vi "FlatToRichcif_plugincore_PluginNames.vi"(5 "OutputClusterType":T1, 11 "InputCluster":T2) -> (3 "OutputCluster":T1)   [LabVIEW 2021, in "CIF_Manager_server.lvlib"]
uses:
  CIF_Manager_server.lvlib
  cif_plugincore_PluginNames_Flat.ctl
  cif_plugincore_PluginNames.ctl
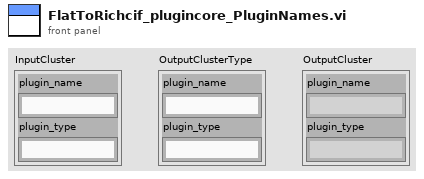
[diagram p1: front panel]
types:
  T1 = typedef "CIF_Manager_server.lvlib/cif_plugincore_PluginNames.ctl" = cluster{"plugin_name":string, "plugin_type":string}
  T2 = typedef "CIF_Manager_server.lvlib/cif_plugincore_PluginNames_Flat.ctl" = cluster{"plugin_name":string, "plugin_type":string}
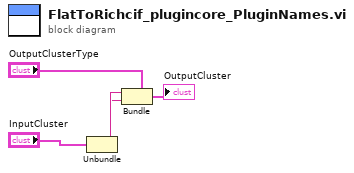
[diagram p0: block diagram]
diagram:
  n1 = Unbundle "Unbundle"("InputCluster") -> ("plugin_name"=w2:string, "plugin_type"=w1:string)
  n2 = Bundle "Bundle"(cluster="OutputClusterType", "plugin_name"=w2, "plugin_type"=w1) -> (→"OutputCluster":T1)
